vi "test-TimeInterpBoolean-Test1.vi"() -> (3 "All tests passed":bool)   [LabVIEW 2019]
uses:
  <vilib>/Rock Robotics/WPI/ThirdParty/JAS_Junk/TrajLib/TIME_INTERPOLATABLE_BOOLEAN.ctl
  <vilib>/Rock Robotics/WPI/ThirdParty/JAS_Junk/TrajLib/TimeInterpBoolean_CleanUp.vi
  <vilib>/gmath/interp.llb/Search Ordered Table.vi
  <vilib>/Rock Robotics/WPI/ThirdParty/JAS_Junk/TrajLib/Trajectory_Library.lvlib
panel:
  out "out TimeInterpBoolean 2":T1
  out "out TimeInterpBoolean":T1
  out "T 11":bool
  out "T 10":bool
  out "T 9":bool
  out "T 8":bool
  out "T 7":bool
  out "T 6":bool
  out "T 5":bool
  out "T 4":bool
  out "T 3":bool
  out "T 2":bool
  out "T 1":bool
  out "T 0":bool
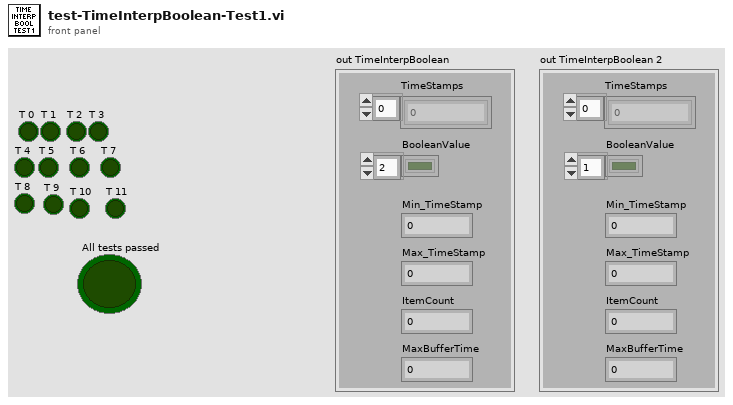
[diagram p1: front panel]
types:
  T1 = typedef "Trajectory_Library.lvlib/TIME_INTERPOLATABLE_BOOLEAN.ctl" = cluster{"TimeStamps":dbl[], "BooleanValue":bool[], "Min_TimeStamp":dbl, "Max_TimeStamp":dbl, "ItemCount":i32, "MaxBufferTime":dbl}
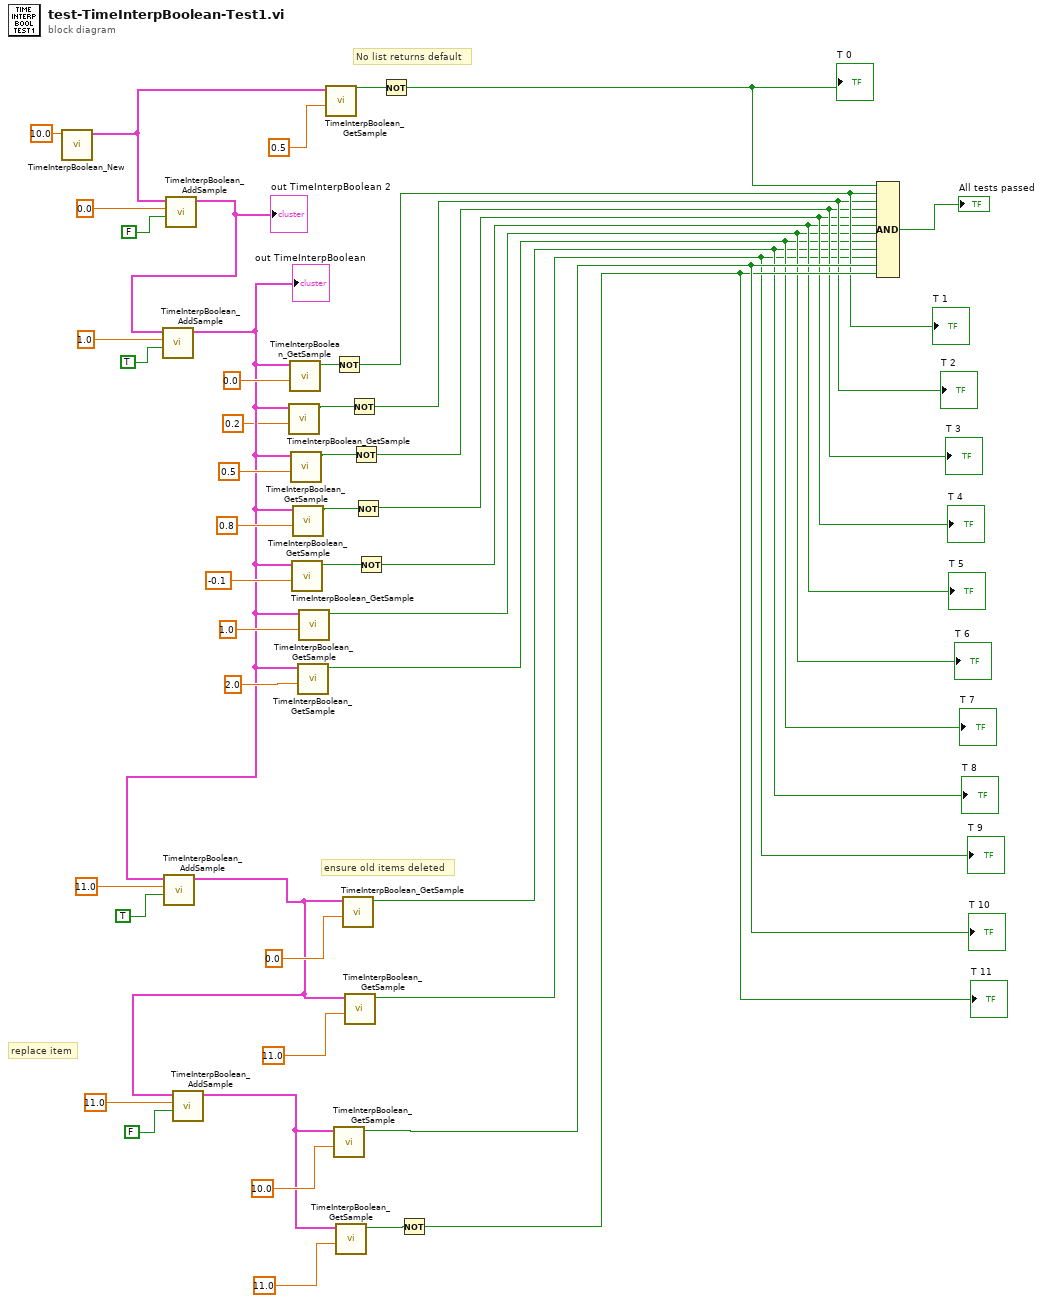
[diagram p0: block diagram]
diagram:
  # "replace item"
  # "ensure old items deleted"
  # "No list returns default"
  n1 = call <vilib>:"TimeInterpBoolean_New.vi"("MaxTime"=10.0) -> ("TimeInterpBoolean"=w39:T1)  [unwired: 10 in]
  n2 = call <vilib>:"TimeInterpBoolean_AddSample.vi"("Value"=FALSE, "TimeStamp"=0.0, "in TimeInterpBoolean"=w39) -> ("out TimeInterpBoolean"=w40:T1)  [unwired: 7 in, 1 out]
  "out TimeInterpBoolean 2" <- w40
  n3 = call <vilib>:"TimeInterpBoolean_AddSample.vi"("Value"=TRUE, "TimeStamp"=1.0, "in TimeInterpBoolean"=w40) -> ("out TimeInterpBoolean"=w20:T1)  [unwired: 7 in, 1 out]
  "out TimeInterpBoolean" <- w20
  n4 = call <vilib>:"TimeInterpBoolean_AddSample.vi"("Value"=TRUE, "TimeStamp"=11.0, "in TimeInterpBoolean"=w20) -> ("out TimeInterpBoolean"=w16:T1)  [unwired: 7 in, 1 out]
  n5 = call <vilib>:"TimeInterpBoolean_AddSample.vi"("Value"=FALSE, "TimeStamp"=11.0, "in TimeInterpBoolean"=w16) -> ("out TimeInterpBoolean"=w13:T1)  [unwired: 7 in, 1 out]
  n6 = call <vilib>:"TimeInterpBoolean_GetSample.vi"("TimeStamp"=0.2, "TimeInterpBoolean"=w20) -> ("OutputBoolean"=w21:bool)  [unwired: 9 in]
  n7 = call <vilib>:"TimeInterpBoolean_GetSample.vi"("TimeStamp"=0.0, "TimeInterpBoolean"=w20) -> ("OutputBoolean"=w25:bool)  [unwired: 9 in]
  n8 = call <vilib>:"TimeInterpBoolean_GetSample.vi"("TimeStamp"=0.5, "TimeInterpBoolean"=w20) -> ("OutputBoolean"=w29:bool)  [unwired: 9 in]
  n9 = call <vilib>:"TimeInterpBoolean_GetSample.vi"("TimeStamp"=-0.1, "TimeInterpBoolean"=w20) -> ("OutputBoolean"=w28:bool)  [unwired: 9 in]
  n10 = call <vilib>:"TimeInterpBoolean_GetSample.vi"("TimeStamp"=0.8, "TimeInterpBoolean"=w20) -> ("OutputBoolean"=w23:bool)  [unwired: 9 in]
  n11 = call <vilib>:"TimeInterpBoolean_GetSample.vi"("TimeStamp"=2.0, "TimeInterpBoolean"=w20) -> ("OutputBoolean"=w3:bool)  [unwired: 9 in]
  "T 7" <- w3
  n12 = call <vilib>:"TimeInterpBoolean_GetSample.vi"("TimeStamp"=1.0, "TimeInterpBoolean"=w20) -> ("OutputBoolean"=w4:bool)  [unwired: 9 in]
  "T 6" <- w4
  n13 = call <vilib>:"TimeInterpBoolean_GetSample.vi"("TimeStamp"=0.5, "TimeInterpBoolean"=w39) -> ("OutputBoolean"=w33:bool)  [unwired: 9 in]
  n14 = Not(x=w25) -> (.not. x?=w9:bool)
  "T 1" <- w9
  n15 = call <vilib>:"TimeInterpBoolean_GetSample.vi"("TimeStamp"=10.0, "TimeInterpBoolean"=w13) -> ("OutputBoolean"=w11:bool)  [unwired: 9 in]
  "T 10" <- w11
  n16 = call <vilib>:"TimeInterpBoolean_GetSample.vi"("TimeStamp"=11.0, "TimeInterpBoolean"=w13) -> ("OutputBoolean"=w12:bool)  [unwired: 9 in]
  n17 = call <vilib>:"TimeInterpBoolean_GetSample.vi"("TimeStamp"=0.0, "TimeInterpBoolean"=w16) -> ("OutputBoolean"=w2:bool)  [unwired: 9 in]
  "T 8" <- w2
  n18 = call <vilib>:"TimeInterpBoolean_GetSample.vi"("TimeStamp"=11.0, "TimeInterpBoolean"=w16) -> ("OutputBoolean"=w1:bool)  [unwired: 9 in]
  "T 9" <- w1
  n19 = Not(x=w21) -> (.not. x?=w8:bool)
  "T 2" <- w8
  n20 = Not(x=w29) -> (.not. x?=w7:bool)
  "T 3" <- w7
  n21 = Not(x=w23) -> (.not. x?=w6:bool)
  "T 4" <- w6
  n22 = Not(x=w28) -> (.not. x?=w5:bool)
  "T 5" <- w5
  n23 = Not(x=w33) -> (.not. x?=w32:bool)
  "T 0" <- w32
  n24 = Not(x=w12) -> (.not. x?=w10:bool)
  "T 11" <- w10
  n25 = Compound Arithmetic op=AND(w32, w9, w8, w7, w6, w5, w4, w3, w2, w1, w11, w10) -> (→"All tests passed":bool)
